vi "PID Climb (Arms Down).vi"(8 "R Sensor Position":dbl, 11 "L Sensor Position":dbl) -> (0 "R Motor Output":dbl, 3 "L Motor Output":dbl)   [LabVIEW 2019]
uses:
  <vilib>/addons/control/pid/NI_PID_pid.lvlib
  <vilib>/addons/control/pid/pid.llb/PID (DBL).vi
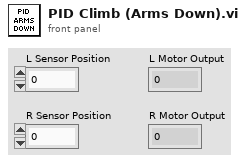
[diagram p1: front panel]
types:
  T1 = cluster{"proportional gain (Kc)":dbl, "integral time (Ti, min)":dbl, "derivative time (Td, min)":dbl}
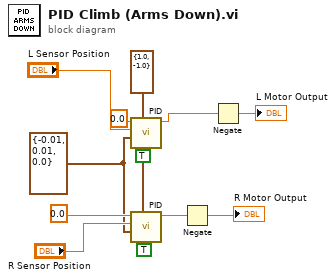
[diagram p0: block diagram]
diagram:
  w1 = T1 {"proportional gain (Kc)"=-0.01, "integral time (Ti, min)"=0.01, "derivative time (Td, min)"=0.0} ("PID gains")
  w6 = cluster{"output high":dbl, "output low":dbl} {"output high"=1.0, "output low"=-1.0} ("output range")
  n1 = call-poly <vilib>:"PID.vi"("reinitialize? (F)"=TRUE, "output range"=w6, "PID gains"=w1, "process variable"="L Sensor Position", "setpoint"=0.0) -> ("output"=w11:dbl)  [unwired: 5 in, 1 out]
  n2 = call-poly <vilib>:"PID.vi"("reinitialize? (F)"=TRUE, "output range"=w6, "PID gains"=w1, "process variable"="R Sensor Position", "setpoint"=0.0) -> ("output"=w10:dbl)  [unwired: 5 in, 1 out]
  n3 = Negate(x=w10) -> (-x=→"R Motor Output":dbl)
  n4 = Negate(x=w11) -> (-x=→"L Motor Output":dbl)
